vi "Main Read Incoming Messages.vi"(8 "error in":errorcluster, 11 "internal data":T1={"J1939 XNET Settings"={"XNET Database"="", "XNET Cluster"="", "CAN port"="", "Baud rate [Bd]"=0, "J1939 Network Address"=0, "Name"=0, "Termination"=0}, "j1939 queues"={"Processed Outgoing"=refnum, "Process Outgoing"=refnum, "stop notifier"=refnum, "error queue"=refnum, "active dtc"=refnum, "processed inc"=refnum}, "fgv references"={"BAM Buffer"=refnum, "CM Buffer"=refnum, "CM Gen"=refnum, "BAM Gen"=refnum, "Address Claims"=refnum, "RQST"=refnum, "scaling lut"=refnum, "data lut"=refnum, "cyclic scheduler"=refnum}, "frame in"="", "frame out"="", "timing"={"tb to j1939 queue timeout"=100, "j1939 to tb queue timeout"=100, "dtc loop period (ms)"=100, "CAN in loop period (ms)"=100, "process incoming queue timeout (ms)"=100, "Outgoing Write Decimation"=0, "process outgoing loop rate (ms)"=0, "periodic outgoing queue timeout (ms)"=10, "CAN out queue timeout (ms)"=100}}) -> ()   [LabVIEW 2013, in "J1939.lvlib"]
uses:
  J1939.lvlib
  API Types/Internal Data.ctl
  API Types/XNET Settings.ctl
  API Types/Setup Information Cluster.ctl
  API Types/CAN Outgoing Message Cluster.ctl
  API Types/Convert DTCs Cluster.ctl
  <vilib>/xnet/xnet.llb/XNET Frame CAN.ctl
  <vilib>/xnet/xnet.llb/XNET Frame Type CAN.ctl
  TP/TP List References.ctl
  BAM/BAM Buffer Connections List_Ref.ctl
  Connection Mode/Connection Mode Generation Connection Ref.ctl
  BAM/BAM Generation Connections List_Ref.ctl
  LUTs/J1939 Address Table Reference.ctl
  RQST/RQST Lookup Table Reference.ctl
  LUTs/J1939 Conversion Lookup Table Reference.ctl
  LUTs/J1939 Data Lookup Table Reference.ctl
  LUTs/Cyclic Frame Scheduler Lut Reference.ctl
  Configuration/TypeDefs/timing configuration.ctl
  Filter by Device Address.vi
  Process Incoming Messages by PDU F.vi
  BAM/BAM Buffer.vi
  TP/TP Buffer Check Timeout on Connections.vi
  Buffer Connections List_Actions.vi
  Connection Mode/Connnection Mode Buffer.vi
  Common Messages/J1939 Message TP.Conn Abort.vi
  Parse Message Type.vi
  RQST/RQST Lookup Table Act.vi
  Frame Conversion/Common Conversions.vi
  Frame Conversion/Convert CAN Arb ID to J1939 ID.vi
  Frame Conversion/Convert J1939 ID to CAN Arb ID.vi
  Frame Conversion/Convert CAN Data (U32) to U8.vi
  Convert Signals to Frame by ID.vi
  Common Messages/J1939 Common Messages.vi
  Common Messages/J1939 Message Acknowledgement.vi
  TP/TP Buffer Search for Connection (No PGN).vi
  TP/TP Buffer Add New Data Packet to Connection.vi
  TP/TP Buffer Convert Connection Info to CAN Frame.vi
  TP/TP Buffer Create New TP Connection.vi
  Common Messages/J1939 Message TP.CM EndofMsgACK.vi
  Common Messages/J1939 Message TP.CM CTS.vi
  Connection Mode/Connection Mode Generation.vi
  Connection Mode/Connection Mode Generation Connections List_Actions.vi
  Connection Mode/Connection Mode Generation Search for Connection (Remote Message).vi
  TP/TP Buffer Search for Connection.vi
  Connection Mode/Connection Mode Generation CTS Received.vi
  LUTs/J1939 Network Address Lookup Table.vi
  Conversion Lookup Table Get Conversion Parameter.vi
  LUTs/J1939 Data Lookup Table Get Signals (Range).vi
  Frame Conversion/Convert PGN + SA to J1939 ID.vi
  <vilib>/xnet/xnet.llb/XNET Read (Frame CAN).vi
  <vilib>/xnet/xnet.llb/XNET Convert.vi
  <vilib>/xnet/xnet.llb/XNET Convert (Signal to Frame Raw).vi
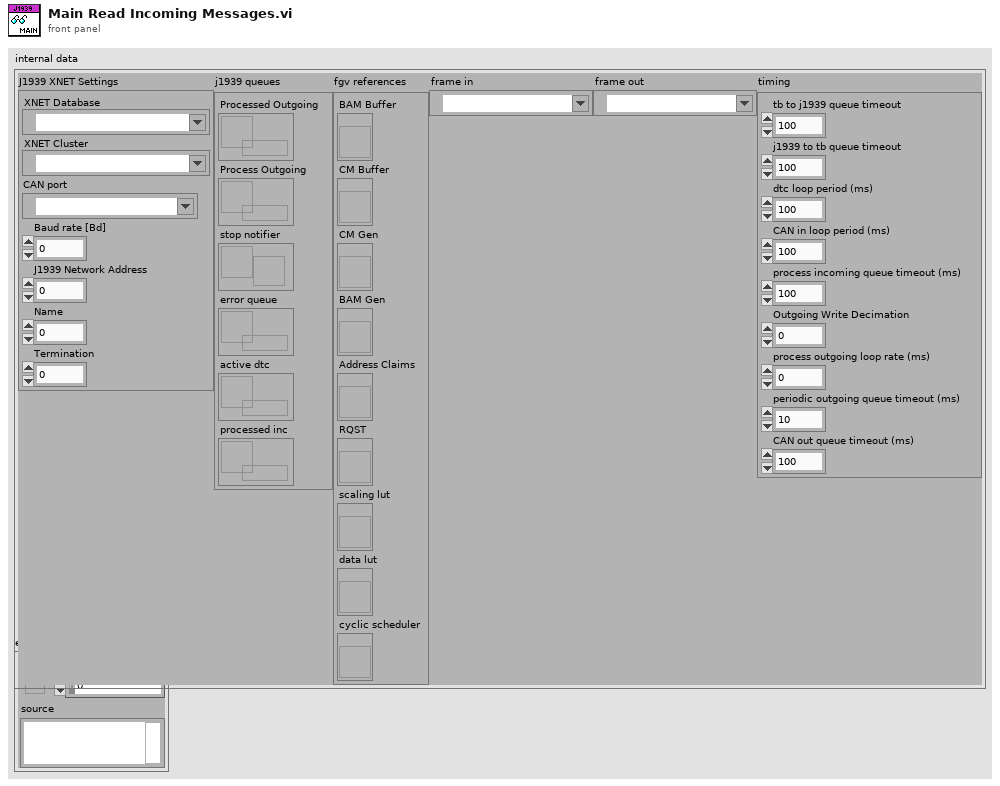
[diagram p1: front panel]
types:
  T1 = typedef "J1939.lvlib/Internal Data.ctl" = cluster{"J1939 XNET Settings":T2, "j1939 queues":T3, "fgv references":T4, "frame in":refnum<k21>, "frame out":refnum<k21>, "timing":T13}
  T2 = typedef "J1939.lvlib/XNET settings.ctl" = cluster{"XNET Database":refnum<k21>, "XNET Cluster":refnum<k21>, "CAN port":refnum<k21>, "Baud rate [Bd]":u32, "J1939 Network Address":u8, "Name":u64, "Termination":u32}
  T3 = typedef "J1939.lvlib/Setup Information Cluster.ctl" = cluster{"Processed Outgoing":refnum<queue>, "Process Outgoing":refnum<queue>, "stop notifier":refnum<notifier>, "error queue":refnum<queue>, "active dtc":refnum<queue>, "processed inc":refnum<queue>}
  T4 = typedef "J1939.lvlib/TP List References.ctl" = cluster{"BAM Buffer":T5, "CM Buffer":T5, "CM Gen":T6, "BAM Gen":T7, "Address Claims":T8, "RQST":T9, "scaling lut":T10, "data lut":T11, "cyclic scheduler":T12}
  T5 = typedef "J1939.lvlib/BAM Buffer Connections List_Ref.ctl" = refnum<vi>
  T6 = typedef "J1939.lvlib/Connection Mode Generation Connection Ref.ctl" = refnum<vi>
  T7 = typedef "J1939.lvlib/BAM Generation Connections List_Ref.ctl" = refnum<vi>
  T8 = typedef "J1939.lvlib/J1939 Address Table Reference.ctl" = refnum<vi>
  T9 = typedef "J1939.lvlib/RQST Lookup Table Reference.ctl" = refnum<vi>
  T10 = typedef "J1939.lvlib/J1939 Conversion Lookup Table Reference.ctl" = refnum<vi>
  T11 = typedef "J1939.lvlib/J1939 Data Lookup Table Reference.ctl" = refnum<vi>
  T12 = typedef "J1939.lvlib/cyclic frame scheduler lut reference.ctl" = refnum<vi>
  T13 = typedef "J1939.lvlib/timing configuration.ctl" = cluster{"tb to j1939 queue timeout":i32, "j1939 to tb queue timeout":i32, "dtc loop period (ms)":i32, "CAN in loop period (ms)":i32, "process incoming queue timeout (ms)":i32, "Outgoing Write Decimation":u32, "process outgoing loop rate (ms)":i32, "periodic outgoing queue timeout (ms)":i32, "CAN out queue timeout (ms)":i32}
  T14 = typedef "XNET Frame CAN.ctl" = cluster{"timestamp":timestamp, "payload":u8[], "identifier":u32, "type":T15, "extended?":bool, "echo?":bool}
  T15 = typedef "XNET Frame Type CAN.ctl" = u8
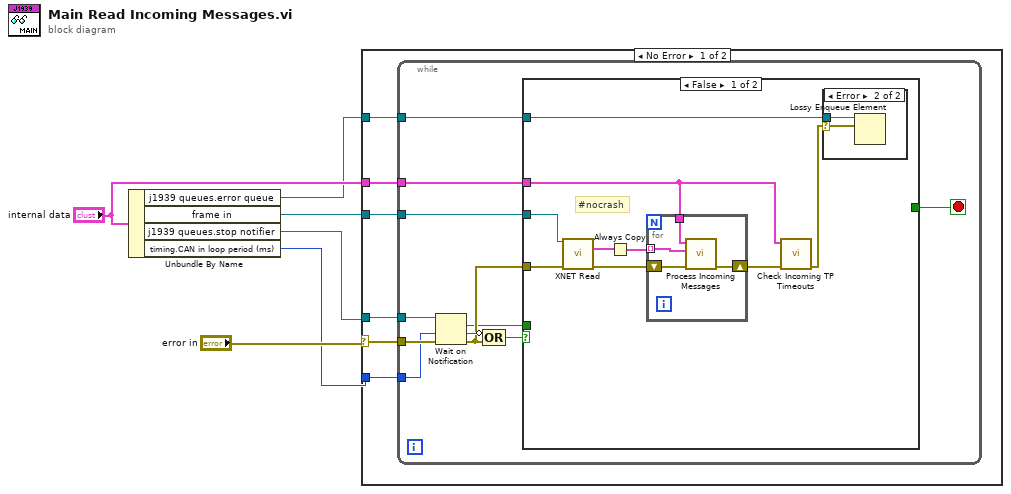
[diagram p0: block diagram]
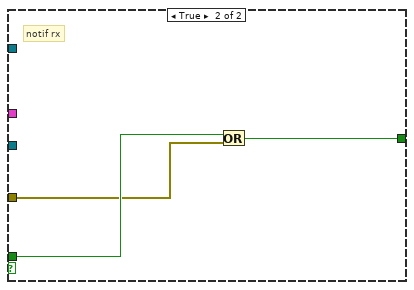
[diagram p3: hidden frame]
diagram:
  n1 = Unbundle By Name("internal data") -> ("j1939 queues.error queue"=w2:refnum<queue>, "frame in"=w5:refnum<k21>, "j1939 queues.stop notifier"=w3:refnum<notifier>, "timing.CAN in loop period (ms)"=w1:i32)
  n2 = case shown="No Error" "error in" {
    selector: "error in" -> [w12 _]
    tunnel: w3 -> [w11 _]
    tunnel: w1 -> [w10 _]
    tunnel: w5 -> [w9 _]
    tunnel: "internal data" -> [w8 _]
    tunnel: w2 -> [w7 _]
    frame No Error {
      n3 = while {
        tunnel: w11 -> [w22]
        tunnel: w12 -> [w23]
        tunnel: w10 -> [w16]
        tunnel: w9 -> [w15]
        tunnel: w8 -> [w14]
        tunnel: w7 -> [w13]
        stop <- w17 stop-if-true
        n4 = Wait on Notification(notifier=w22, timeout in ms (-1)=w16, error in (no error)=w23) -> (notification=w18:bool, timed out?=w21:bool, error out=w19:errorcluster)  [unwired: 1 in, 1 out]
        n5 = Compound Arithmetic op=OR(invert w21, w19) -> (w20:bool)
        n6 = case shown="False" w20 {
          tunnel: w19 -> [w32 w39]
          tunnel: w18 -> [_ w41]
          tunnel: [_ w40] -> w17
          tunnel: w15 -> [w29 _]
          tunnel: w14 -> [w28 _]
          tunnel: w13 -> [w26 _]
          frame False {
            # "#nocrash"
            n7 = call-poly <vilib>:"XNET Read.vi"("session in"=w29, "error in (no error)"=w32) -> ("data"=w30:T14[], "error out"=w31:errorcluster)  [unwired: 12 out]
            n8 = Always Copy(1:w30) -> (0:w24:T14[])
            n9 = for {
              tunnel: w24 -> [w36] mode=indexing
              shift-right: [w34] -> w25
              shift-left: w31 -> [w35]
              tunnel: w28 -> [w33]
              n10 = call "Process Incoming Messages.vi"("error in"=w35, "CAN frame"=w36, "internal data"=w33) -> ("error out"=w34:errorcluster)  [unwired: 8 in]
            }
            n11 = call "Check Incoming TP Timeouts.vi"("error in"=w25, "internal data"=w28) -> ("error out"=w27:errorcluster)  [unwired: 9 in]
            n12 = case shown="Error" w27 {
              selector: w27 -> [_ w38]
              tunnel: w26 -> [_ w37]
              frame No Error {
              }
              frame Error {
                n13 = Lossy Enqueue Element(queue=w37, element=w38) -> ()  [unwired: 1 in, 4 out]
              }
            }
          }
          frame True {
            # "notif rx"
            n14 = Or(x=w41, y=w39) -> (x .or. y?=w40:bool)
          }
        }
      }
    }
    frame Error {
    }
  }
